vi "CreatePicture(TRACE).vi"(9 "plot color":u32, 10 "output cluster 2":T1, 11 "picture in":picture) -> (3 "new picture":picture)   [LabVIEW 2011]
uses:
  scopeTrace_TupDef.ctl
  <vilib>/picture/cartesn2.llb/Waveform Plot Type.ctl
panel:
  out "info Cluster 2":cluster{"t0":dbl, "dt":dbl, "gain":dbl}
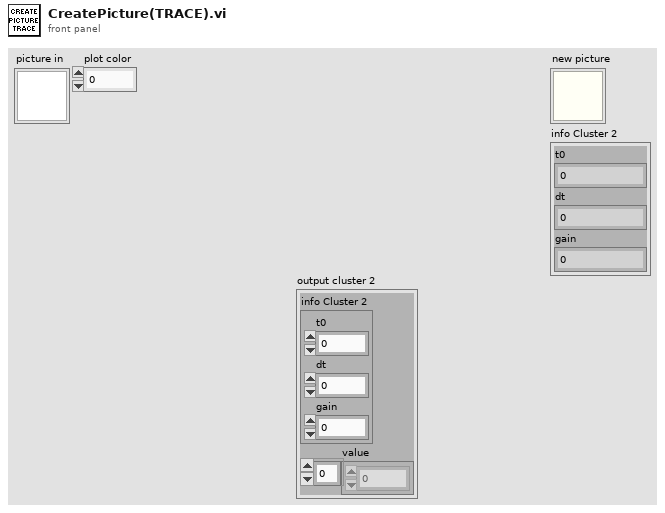
[diagram p1: front panel]
types:
  T1 = typedef "scopeTrace_TupDef.ctl" = cluster{"info Cluster 2":cluster{"t0":dbl, "dt":dbl, "gain":dbl}, "value":i16[]}
  T2 = cluster{"bar width(50%)":dbl, "frame?(T)":bool, "frame color(black)":u32}
  T3 = cluster{"left":i16, "top":i16, "right":i16, "bottom":i16}
  T4 = cluster{"line color":u32, "text color":u32, "tick length(3)":i16, "crossing axes":bool, "visible grid?":bool}
  T5 = enum8{"Decimal", "Scientific", "Engineering", "Binary", "Octal", "Hex"}
  T6 = cluster{"x minimum":dbl, "x maximum":dbl, "x log?":bool, "x precision":u8, "x format":enum8{"Decimal", "Scientific", "Engineering", "Binary", "Octal", "Hex"}, "y minimum":dbl, "y maximum":dbl, "y log?":bool, "y precision":u8, "y format":enum8{"Decimal", "Scientific", "Engineering", "Binary", "Octal", "Hex"}}
  T7 = typedef "Waveform Plot Type.ctl" = enum16{"points", "squares", "circles", "connected points", "connected squares", "connected circles", "fill to baseline", "comb plot", "bar plot"}
  T8 = cluster{"plot color":u32, "waveform plot type":T7, "baseline":dbl}
  T9 = cluster{"Xo(0)":dbl, "delta X(1)":dbl, "Y data":dbl[]}
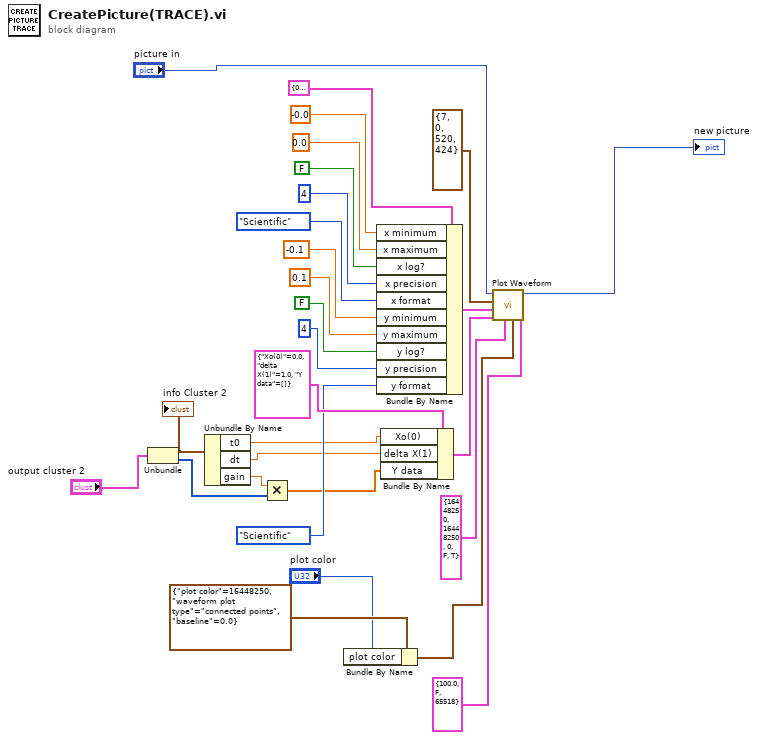
[diagram p0: block diagram]
diagram:
  n1 = Unbundle("output cluster 2") -> ("info Cluster 2"=w6:cluster{"t0":dbl, "dt":dbl, "gain":dbl}, "value"=w4:i16[])
  "info Cluster 2" <- w6
  n2 = Unbundle By Name(w6) -> ("t0"=w1:dbl, "dt"=w2:dbl, "gain"=w5:dbl)
  n3 = Multiply(x=w5, y=w4) -> (x*y=w3:dbl[])
  n4 = Bundle By Name(cluster=T8 {"plot color"=16448250, "waveform plot type"=enum."connected points", "baseline"=0.0} ("waveform plot cosmetics"), "plot color"="plot color") -> (w11:T8)
  n5 = Bundle By Name(cluster=T6 {"x minimum"=0.0, "x maximum"=0.0, "x log?"=FALSE, "x precision"=1, "x format"=enum."Decimal", "y minimum"=0.0, "y maximum"=0.0, "y log?"=FALSE, "y precision"=1, "y format"=enum."Decimal"} ("cartesian axis attributes"), "x minimum"=-0.0, "x maximum"=0.0, "x log?"=FALSE, "x precision"=u8 4, "x format"=T5."Scientific", "y minimum"=-0.1, "y maximum"=0.1, "y log?"=FALSE, "y precision"=u8 4, "y format"=T5."Scientific") -> (w22:T6)
  n6 = Bundle By Name(cluster=T9 {"Xo(0)"=0.0, "delta X(1)"=1.0, "Y data"=[]} ("waveform data"), "Xo(0)"=w1, "delta X(1)"=w2, "Y data"=w3) -> (w13:T9)
  n7 = call <vilib>:"Plot Waveform.vi"("[bar style]"=T2 {"bar width(50%)"=100.0, "frame?(T)"=FALSE, "frame color(black)"=65518}, "waveform plot cosmetics"=w11, "cartesian grid cosmetics"=T4 {"line color"=16448250, "text color"=16448250, "tick length(3)"=0, "crossing axes"=FALSE, "visible grid?"=TRUE}, "waveform data"=w13, "cartesian axis attributes"=w22, "bounding rect"=T3 {"left"=7, "top"=0, "right"=520, "bottom"=424}, "picture"="picture in") -> ("new picture"=→"new picture":picture)  [unwired: 4 in]
